vi "2차원 배열 만들기.vi"() -> ()   [LabVIEW 2017]
uses:
  <vilib>/measure/NI_MABase.lvlib
panel:
  out "Array":dbl[](array[numeric])
  out "Waveform Graph":waveform(dbl)(graph)
  in  "Step":dbl=0.1
  in  "Stop (V)":dbl=2.0
  in  "Start (V)":dbl=1.0
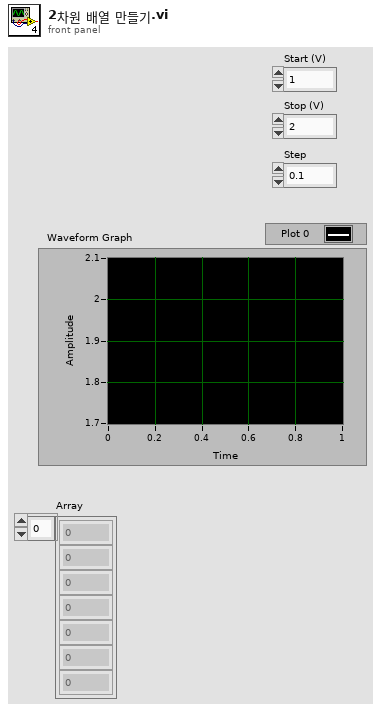
[diagram p1: front panel]
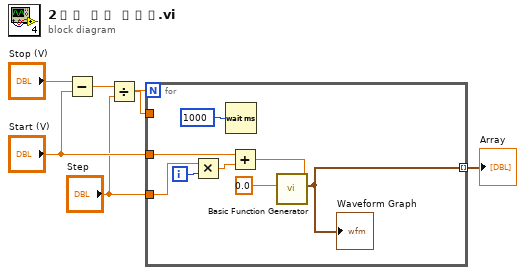
[diagram p0: block diagram]
diagram:
  n1 = Subtract(x="Stop (V)", y="Start (V)") -> (x-y=w6:dbl)
  n2 = Divide(x=w6, y="Step") -> (x/y=w3:dbl)
  n3 = for {
    N: w3 -> [_]
    tunnel: "Start (V)" -> [w13]
    tunnel: w3 -> [_]
    tunnel: "Step" -> [w9]
    tunnel: [w7] -> w1 mode=indexing
    i -> [w12]
    n4 = Multiply(x=w9, y=w12) -> (x*y=w11:dbl)
    n5 = Wait (ms)(milliseconds to wait=u32 1000) -> ()  [unwired: 1 out]
    n6 = Add(x=w13, y=w11) -> (x+y=w14:dbl)
    n7 = call <vilib>:"Basic Function Generator.vi"("offset"=w14, "amplitude"=0.0) -> ("signal out"=w7:waveform(dbl))  [unwired: 7 in, 2 out]
    "Waveform Graph" <- w7
  }
  "Array" <- w1
